vi "CRYPlot Intensity Graph Preview.vi"(10 "sOption":string, 11 "IntensityGraph VI Ref":refnum<vi>) -> ()   [LabVIEW 2013]
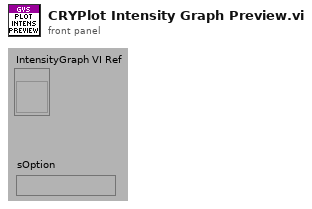
[diagram p1: front panel]
types:
  T1 = typedef "CRYWaveform Cluster.ctl" = cluster{"Waveform":cluster{"X0":dbl, "dX":dbl, "Y":sgl[]}, "X data":u16, "Y data":u16, "Y axis":u16, "X unit":string, "Y unit":string, "Y dB ref":dbl, "display Y":bool, "display X":bool, "Overload?":bool, "Test Info":string, "Step No.":i32, "Name":string, "protected":bool, "Sqc history":string[], "Signal Channel ID":i32, "Plot Settings":cluster{"Color":u32, "Interpolation":u8, "Point Style":u8, "Line Style":u8, "Point Color":u32, "Line Width":u8, "Bar Plot Style":u8, "Fill To":i16}, "AutoProtect":bool}
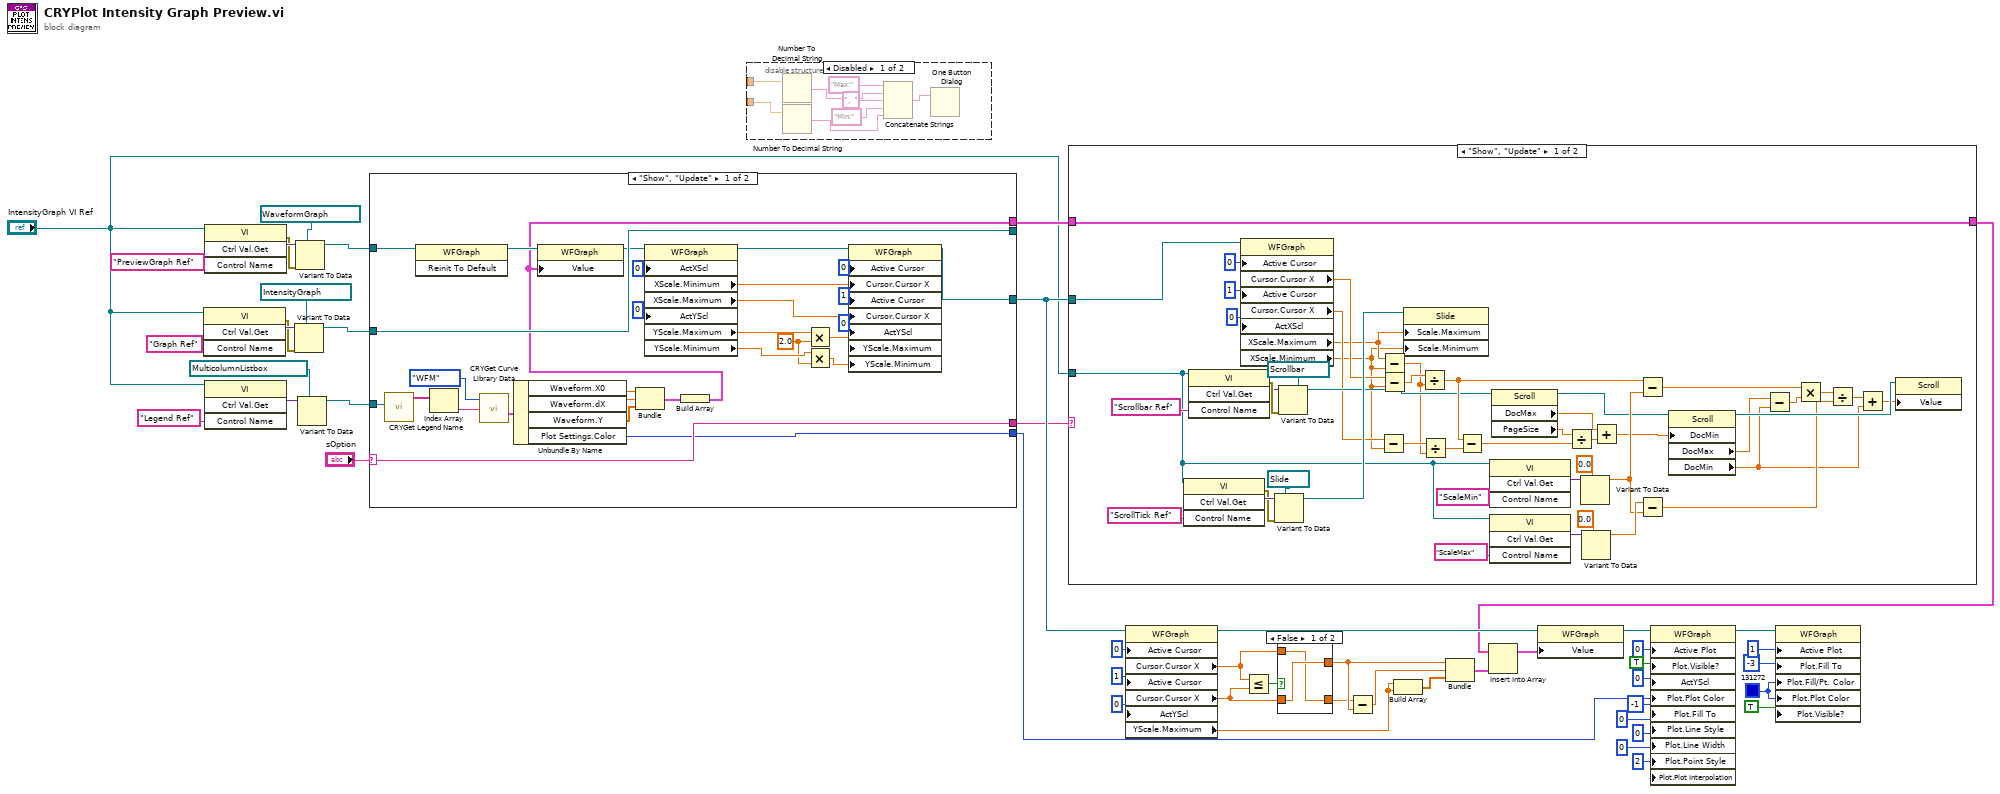
[diagram p0: block diagram]
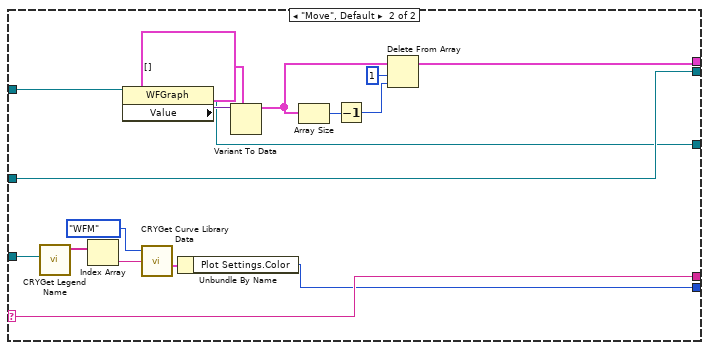
[diagram p5: hidden frame]
diagram:
  w28 = u32 131272
  n1 = invoke class="VI" method="Ctrl Val.Get"(reference="IntensityGraph VI Ref", "Control Name"="Graph Ref") -> (error out=w43:errorcluster, "Get Control Value Variant"=w45:variant)  [unwired: 2 in, 2 out]
  n2 = invoke class="VI" method="Ctrl Val.Get"(reference="IntensityGraph VI Ref", "Control Name"="PreviewGraph Ref") -> (error out=w48:errorcluster, "Get Control Value Variant"=w49:variant)  [unwired: 2 in, 2 out]
  n3 = invoke class="VI" method="Ctrl Val.Get"(reference="IntensityGraph VI Ref", "Control Name"="Legend Ref") -> ("Get Control Value Variant"=w16:variant)  [unwired: 2 in, 3 out]
  n4 = Variant To Data(error in=w43, type=refnum<vi> refnum ("Legend Ref"), Variant=w45) -> (data=w42:refnum<vi>)  [unwired: 1 out]
  n5 = Variant To Data(error in=w48, type=refnum<vi> refnum ("Legend Ref"), Variant=w49) -> (data=w41:refnum<vi>)  [unwired: 1 out]
  n6 = Variant To Data(type=refnum<vi> refnum ("GMListbox"), Variant=w16) -> (data=w13:refnum<vi>)  [unwired: 1 in, 1 out]
  n7 = case shown="\"Show\", \"Update\"" "sOption" {
    selector: "sOption" -> [w66 w87]
    tunnel: w41 -> [w79 w89]
    tunnel: w42 -> [w54 w96]
    tunnel: [w68 w88] -> w39
    tunnel: [w54 w96] -> _
    tunnel: [w51 w86] -> w20
    tunnel: [w66 w87] -> w38
    tunnel: w13 -> [w60 w81]
    tunnel: [w52 w80] -> w2
    frame "Show", "Update" {
      w69 = 2.0 ("y")
      n8 = call "CRYGet Legend Name.vi"("MCListbox Refnum"=w60) -> ("Names Out"=w62:string[])  [unwired: 10 in]
      n9 = invoke class="WFGraph" method="Reinit To Default"(reference=w79) -> (reference out=w67:refnum<vi>)  [unwired: 2 in, 2 out]
      n10 = Index Array(array=w62) -> (element=w61:string)  [unwired: 1 in]
      n11 = call "CRYGet Curve Library Data.vi"("Type"=enum16{"Curves", "Values", "Results", "WFM"}."WFM", "Data Name"=w61) -> ("Wave"=w56:T1)  [unwired: 4 out]
      n12 = Unbundle By Name(w56) -> ("Waveform.X0"=w59:dbl, "Waveform.dX"=w58:dbl, "Waveform.Y"=w57:sgl[], "Plot Settings.Color"=w52:u32)
      n13 = Bundle("X0"=w59, "dX"=w58, "Y"=w57) -> (w55:cluster{"X0":dbl, "dX":dbl, "Y":sgl[]})  [unwired: 1 in]
      n14 = Build Array(w55) -> (w51:cluster{"X0":dbl, "dX":dbl, "Y":sgl[]}[])
      n15 = property class="WFGraph"(reference=w67, "Value"=w51) -> (reference out=w50:refnum<vi>)  [unwired: 1 in, 1 out]
      n16 = property on="Property Node" class="WFGraph"(reference=w50, "ActXScl"=0 ("Active Y Scale"), "ActYScl"=0 ("Active Y Scale")) -> (reference out=w53:refnum<vi>, "XScale.Minimum"=w64:dbl, "XScale.Maximum"=w65:dbl, "YScale.Maximum"=w72:dbl, "YScale.Minimum"=w73:dbl)  [unwired: 1 in, 1 out]
      n17 = Multiply(x=w72, y=w69) -> (x*y=w71:dbl)
      n18 = Multiply(x=w73, y=w69) -> (x*y=w70:dbl)
      n19 = property on="Property Node" class="WFGraph"(reference=w53, "Active Cursor"=u32 0, "Cursor.Cursor X"=w64, "Active Cursor"=u32 1, "Cursor.Cursor X"=w65, "ActYScl"=0 ("Active Y Scale"), "YScale.Maximum"=w71, "YScale.Minimum"=w70) -> (reference out=w68:refnum<vi>)  [unwired: 1 in, 1 out]
    }
    frame "Move", Default {
      n20 = call "CRYGet Legend Name.vi"("MCListbox Refnum"=w81) -> ("Names Out"=w84:string[])  [unwired: 10 in]
      n21 = Index Array(array=w84) -> (element=w83:string)  [unwired: 1 in]
      n22 = property class="WFGraph"(reference=w89) -> (reference out=w88:refnum<vi>, "Value"=w94:variant)  [unwired: 1 in, 1 out]
      n23 = call "CRYGet Curve Library Data.vi"("Type"=enum16{"Curves", "Values", "Results", "WFM"}."WFM", "Data Name"=w83) -> ("Wave"=w82:T1)  [unwired: 4 out]
      n24 = Unbundle By Name(w82) -> ("Plot Settings.Color"=w80:u32)
      n25 = Variant To Data(type=cluster{"xo":dbl, "dx":dbl, dbl[]}[] [] ("appended array"), Variant=w94) -> (data=w92:cluster{"xo":dbl, "dx":dbl, dbl[]}[])  [unwired: 1 in, 1 out]
      n26 = Array Size(array=w92) -> (size(s)=w91:i32)
      n27 = Decrement(x=w91) -> (x-1=w90:i32)
      n28 = Delete From Array(array=w92, length=1, index=w90) -> (array with subset deleted=w86:cluster{"xo":dbl, "dx":dbl, dbl[]}[])  [unwired: 1 out]
    }
  }
  n29 = disable-structure shown="Disabled" {
    disable-tunnel: _ -> [w104 _]
    disable-tunnel: _ -> [w103 _]
    frame Disabled {
      n30 = Number To Decimal String(number=w104) -> (decimal integer string=w101:string)  [unwired: 1 in]
      n31 = Number To Decimal String(number=w103) -> (decimal integer string=w98:string)  [unwired: 1 in]
      n32 = Concatenate Strings("Max:" ("string"), w101, ", " ("string"), "Min:" ("string"), w98) -> (w97:string)
      n33 = One Button Dialog(message=w97) -> ()  [unwired: 1 in, 1 out]
    }
    frame Enabled {
    }
  }
  n34 = case shown="\"Show\", \"Update\"" w38 {
    tunnel: "IntensityGraph VI Ref" -> [w110 _]
    tunnel: w39 -> [w109 _]
    tunnel: w20 -> [w105 w153]
    tunnel: [w105 w153] -> w19
    frame "Show", "Update" {
      n35 = invoke class="VI" method="Ctrl Val.Get"(reference=w110, "Control Name"="ScrollTick Ref") -> (error out=w144:errorcluster, "Get Control Value Variant"=w145:variant)  [unwired: 2 in, 2 out]
      n36 = invoke class="VI" method="Ctrl Val.Get"(reference=w110, "Control Name"="Scrollbar Ref") -> (error out=w139:errorcluster, "Get Control Value Variant"=w138:variant)  [unwired: 2 in, 2 out]
      n37 = property on="Property Node" class="WFGraph"(reference=w109, "Active Cursor"=u32 0, "Active Cursor"=u32 1, "ActXScl"=0 ("Active X Scale")) -> ("Cursor.Cursor X"=w112:dbl, "Cursor.Cursor X"=w111:dbl, "XScale.Maximum"=w108:dbl, "XScale.Minimum"=w107:dbl)  [unwired: 1 in, 2 out]
      n38 = Variant To Data(error in=w144, type=refnum<vi> refnum ("Legend Ref"), Variant=w145) -> (data=w147:refnum<vi>)  [unwired: 1 out]
      n39 = Variant To Data(error in=w139, type=refnum<vi> refnum ("Legend Ref"), Variant=w138) -> (data=w141:refnum<vi>)  [unwired: 1 out]
      n40 = Subtract(x=w111, y=w107) -> (x-y=w151:dbl)
      n41 = Subtract(x=w108, y=w107) -> (x-y=w106:dbl)
      n42 = Subtract(x=w112, y=w107) -> (x-y=w149:dbl)
      n43 = property on="Property Node" class="Slide"(reference=w147, "Scale.Maximum"=w108, "Scale.Minimum"=w107) -> ()  [unwired: 1 in, 2 out]
      n44 = Divide(x=w149, y=w106) -> (x/y=w150:dbl)
      n45 = Divide(x=w151, y=w106) -> (x/y=w152:dbl)
      n46 = Subtract(x=w150, y=w152) -> (x-y=w124:dbl)
      n47 = invoke class="VI" method="Ctrl Val.Get"(reference=w110, "Control Name"="ScaleMin") -> ("Get Control Value Variant"=w130:variant)  [unwired: 2 in, 3 out]
      n48 = invoke class="VI" method="Ctrl Val.Get"(reference=w110, "Control Name"="ScaleMax") -> ("Get Control Value Variant"=w133:variant)  [unwired: 2 in, 3 out]
      n49 = property on="Property Node" class="Scroll"(reference=w141) -> (reference out=w126:refnum<vi>, "DocMax"=w122:dbl, "PageSize"=w115:dbl)  [unwired: 1 in, 1 out]
      n50 = Divide(x=w115, y=w124) -> (x/y=w125:dbl)
      n51 = Variant To Data(type=0.0 ("X Scale.Range:Maximum"), Variant=w130) -> (data=w134:dbl)  [unwired: 1 in, 1 out]
      n52 = Variant To Data(type=0.0 ("X Scale.Range:Maximum"), Variant=w133) -> (data=w135:dbl)  [unwired: 1 in, 1 out]
      n53 = Add(x=w122, y=w125) -> (x+y=w123:dbl)
      n54 = Subtract(x=w150, y=w134) -> (x-y=w121:dbl)
      n55 = Subtract(x=w135, y=w134) -> (x-y=w118:dbl)
      n56 = property on="Property Node" class="Scroll"(reference=w126, "DocMin"=w123) -> (reference out=w127:refnum<vi>, "DocMax"=w113:dbl, "DocMin"=w114:dbl)  [unwired: 1 in, 1 out]
      n57 = Subtract(x=w113, y=w114) -> (x-y=w120:dbl)
      n58 = Multiply(x=w121, y=w120) -> (x*y=w119:dbl)
      n59 = Divide(x=w119, y=w118) -> (x/y=w117:dbl)
      n60 = Add(x=w117, y=w114) -> (x+y=w116:dbl)
      n61 = property on="Property Node" class="Scroll"(reference=w127, "Value"=w116) -> ()  [unwired: 1 in, 2 out]
    }
    frame Default {
    }
  }
  n62 = property on="Property Node" class="WFGraph"(reference=w39, "Active Cursor"=u32 0, "Active Cursor"=u32 1, "ActYScl"=0 ("Active Y Scale")) -> (reference out=w31:refnum<vi>, "Cursor.Cursor X"=w25:dbl, "Cursor.Cursor X"=w26:dbl, "YScale.Maximum"=w37:dbl)  [unwired: 1 in, 1 out]
  n63 = Less Or Equal?(x=w25, y=w26) -> (x <= y?=w23:bool)
  n64 = case shown="False" w23 {
    tunnel: [w155 w157] -> w36
    tunnel: w25 -> [w154 w157]
    tunnel: [w154 w156] -> w35
    tunnel: w26 -> [w155 w156]
    frame False {
    }
    frame True {
    }
  }
  n65 = Subtract(x=w35, y=w36) -> (x-y=w32:dbl)
  n66 = Build Array(w37, w37) -> (w33:dbl[])
  n67 = Bundle("Cursor.Cursor X"=w36, w32, w33) -> (w34:cluster{"Cursor.Cursor X":dbl, dbl, dbl[]})  [unwired: 1 in]
  n68 = Insert Into Array(array=w19, new element=w34) -> (w1:cluster{"xo":dbl, "dx":dbl, "Y":dbl[]}[])  [unwired: 1 in]
  n69 = property class="WFGraph"(reference=w31, "Value"=w1) -> (reference out=w18:refnum<vi>)  [unwired: 1 in, 1 out]
  n70 = property class="WFGraph"(reference=w18, "Active Plot"=u32 0, "Plot.Visible?"=TRUE ("Plot.Visible"), "ActYScl"=0 ("Active Y Scale"), "Plot.Plot Color"=w2, "Plot.Fill To"=i16 -1, "Plot.Line Style"=u8 0, "Plot.Line Width"=u8 0, "Plot.Point Style"=u8 0, "Plot.Plot Interpolation"=u8 2) -> (reference out=w24:refnum<vi>)  [unwired: 1 in, 1 out]
  n71 = property on="Property Node" class="WFGraph"(reference=w24, "Active Plot"=u32 1, "Plot.Fill To"=i16 -3, "Plot.Fill/Pt. Color"=w28, "Plot.Plot Color"=w28, "Plot.Visible?"=TRUE ("Plot.Visible")) -> ()  [unwired: 1 in, 2 out]
